vi "maquinadeestadosporsondeo.vi"() -> ()   [LabVIEW 2016]
uses:
  Control 4.ctl
panel:
  in  "Detener":bool
  out "MD":bool
  out "MI":bool
  in  "S":bool
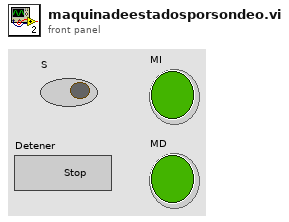
[diagram p1: front panel]
types:
  T1 = typedef "Control 4.ctl" = enum16{"Avance1", "Izquierda", "Derecha", "Paro", "Avance2"}
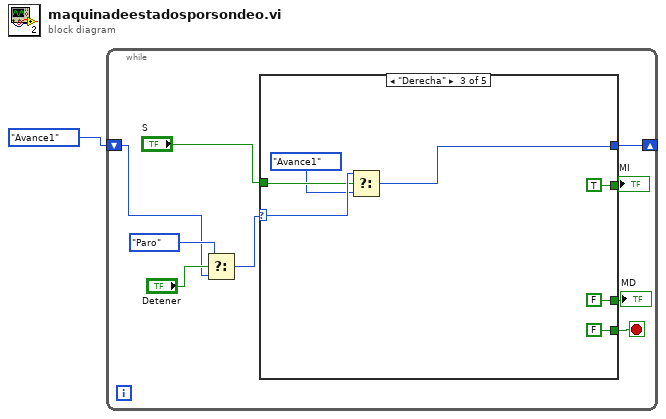
[diagram p0: block diagram]
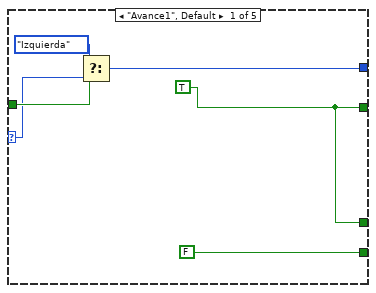
[diagram p2: hidden frame]
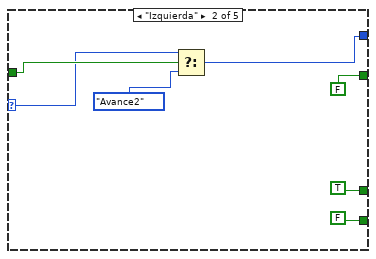
[diagram p3: hidden frame]
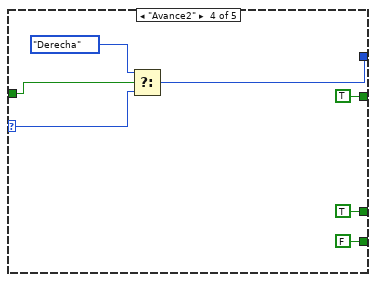
[diagram p4: hidden frame]
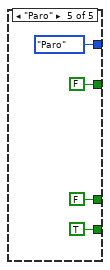
[diagram p5: hidden frame]
diagram:
  n1 = while {
    shift-right: [w6] -> _
    shift-left: Control_4."Avance1" -> [w3]
    stop <- w8 stop-if-true
    n2 = Select(t=Control_4."Paro", s="Detener", f=w3) -> (s? t:f=w2:T1)
    n3 = case shown="\"Derecha\"" w2 {
      selector: w2 -> [w11 w17 w27 w33 _]
      tunnel: [w16 FALSE TRUE TRUE FALSE] -> w10
      tunnel: [w16 TRUE FALSE TRUE FALSE] -> w9
      tunnel: [FALSE FALSE FALSE FALSE TRUE] -> w8
      tunnel: "S" -> [w14 w20 w26 w34 _]
      tunnel: [w12 w18 w24 w31 Control_4."Paro"] -> w6
      frame "Avance1", Default {
        w16 = TRUE
        n4 = Select(t=Control_4."Izquierda", s=w14, f=w11) -> (s? t:f=w12:T1)
      }
      frame "Izquierda" {
        n5 = Select(t=w17, s=w20, f=Control_4."Avance2") -> (s? t:f=w18:T1)
      }
      frame "Derecha" {
        n6 = Select(t=w27, s=w26, f=Control_4."Avance1") -> (s? t:f=w24:T1)
      }
      frame "Avance2" {
        n7 = Select(t=Control_4."Derecha", s=w34, f=w33) -> (s? t:f=w31:T1)
      }
      frame "Paro" {
      }
    }
    "MD" <- w9
    "MI" <- w10
  }
